vi "Logger-Close Log.vi"(11 "error in (no error)":errorcluster) -> (15 "error out":errorcluster)   [LabVIEW 2020]
uses:
  Typedefs/Logger-Queue Data.ctl
  Typedefs/Logger-Action.ctl
  Typedefs/Logger-Level.ctl
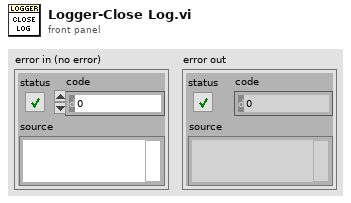
[diagram p1: front panel]
types:
  T1 = typedef "Logger-Queue Data.ctl" = cluster{"Action":T2, "Level":T3, "Time":dbl, "Message":string}
  T2 = typedef "Logger-Action.ctl" = enum16{"None", "Init", "Add", "Show", "Offset", "Quit"}
  T3 = typedef "Logger-Level.ctl" = enum16{"Debug", "TCP", "Info", "Warning", "Error", "Critical"}
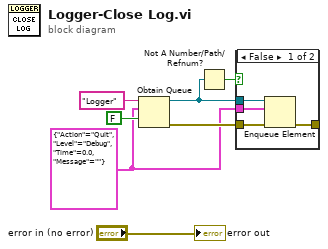
[diagram p0: block diagram]
diagram:
  w1 = T1 {"Action"=enum."Quit", "Level"=enum."Debug", "Time"=0.0, "Message"=""} ("Trace Data")
  n1 = Obtain Queue(name (unnamed)="Logger", element data type=w1, create if not found? (T)=FALSE) -> (queue out=w3:refnum<queue>, error out=w4:errorcluster)  [unwired: 2 in, 1 out]
  n2 = Not A Number/Path/Refnum?(number/path/refnum=w3) -> (NaN/Path/Refnum?=w2:bool)
  n3 = case shown="False" w2 {
    tunnel: w1 -> [w11 _]
    tunnel: w4 -> [w10 _]
    tunnel: w3 -> [w9 _]
    tunnel: [w8 _] -> _
    frame False {
      n4 = Enqueue Element(queue=w9, element=w11, error in (no error)=w10) -> (error out=w8:errorcluster)  [unwired: 1 in, 2 out]
    }
    frame True {
    }
  }
  "error out" <- "error in (no error)"
